vi "Last Ack Created Queue.vi"(10 "Queue":refnum<class "Queue.lvclass">, 11 "jettl Msg Last Ack Created Queue in":refnum<class "jettl Msg Last Ack Created Queue.lvclass">) -> (3 "jettl Msg Last Ack Created Queue out":refnum<class "jettl Msg Last Ack Created Queue.lvclass">)   [LabVIEW 2021, in "jettl.lvlib" / "jettl Msg Last Ack Created Queue.lvlib" / "jettl Msg Last Ack Created Queue.lvclass"]
uses:
  jettl Msg Last Ack Created Queue.lvclass
  Queue/Queue.lvclass
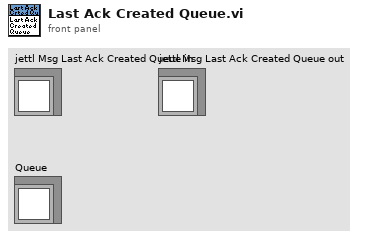
[diagram p1: front panel]
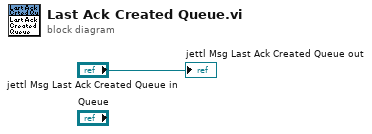
[diagram p0: block diagram]
diagram:
  "jettl Msg Last Ack Created Queue out" <- "jettl Msg Last Ack Created Queue in"
